vi "RELAYS Delay ON a Relay.vi"(6 "delayed Time ( 2 sec)":dbl=2.0, 8 "error in (no error)":errorcluster, 9 "Relays IDs":T1=3 items=["Relay 1"=3, "Relay 2"=8, "Relay 3"=13, "Relay 4"=18, "Relay 5"=23, "Relay 6"=28, "Relay 7"=33, "Relay 8"=38], 10 "Dev addr":u8=1 format="%x", 11 "VISA resource name":refnum<visa-resource-name>) -> (0 "error out":errorcluster, 1 "success?":bool, 2 "ack":string, 3 "VISA resource name out":refnum<visa-resource-name>)   [LabVIEW 2016, in "MB _relays.lvlib"]
uses:
  MB _relays.lvlib
  type defs/Relays IDs flash.ctl
  private/gen MB frame -Delayed ON Relay.vi
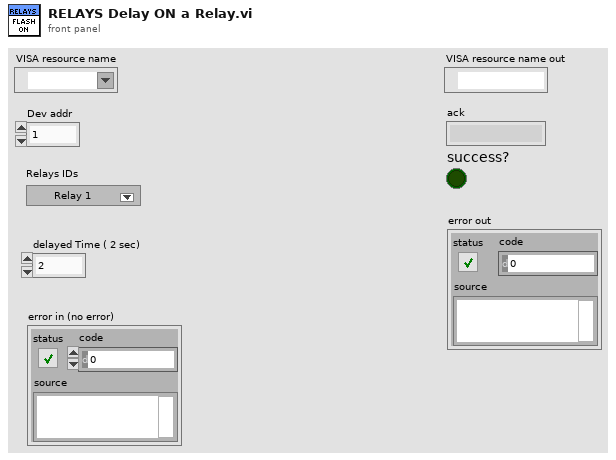
[diagram p1: front panel]
types:
  T1 = typedef "MB _relays.lvlib/Relays IDs flash.ctl" = u16
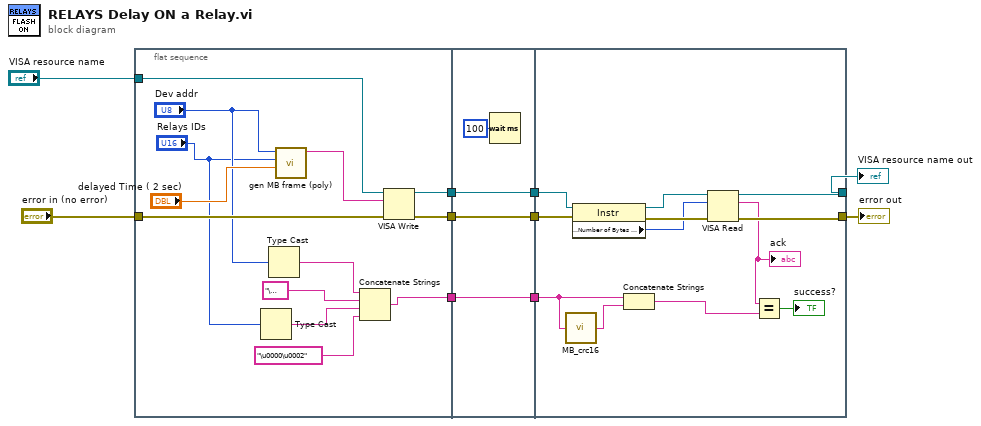
[diagram p0: block diagram]
diagram:
  n1 = flat-sequence {
    tunnel: "error in (no error)" -> [w20]
    tunnel: "VISA resource name" -> [w19]
    tunnel: [w23] -> w6
    tunnel: [w22] -> w5
    tunnel: [w11] -> w2
    tunnel: w6 -> [w27]
    tunnel: w5 -> [w26]
    tunnel: [w27] -> w4
    tunnel: [w26] -> w3
    tunnel: w2 -> [w24]
    tunnel: [w24] -> w1
    tunnel: [w33] -> w9
    tunnel: [w34] -> w10
    tunnel: w4 -> [w38]
    tunnel: w3 -> [w39]
    tunnel: w1 -> [w31]
    frame #0 {
      n2 = Type Cast(x="Relays IDs") -> (*(type *) &x=w13:string)  [unwired: 1 in]
      n3 = Type Cast(x="Dev addr") -> (*(type *) &x=w15:string)  [unwired: 1 in]
      n4 = call-poly "gen MB frame (poly).vi"("Half Period(sec)"="delayed Time ( 2 sec)", "Relays IDs"="Relays IDs", "Dev Addr"="Dev addr") -> ("MB frame"=w21:string)  [unwired: 8 in]
      n5 = Concatenate Strings(w15, "\u0010", w13, "\u0000\u0002") -> (w11:string)
      n6 = VISA Write(VISA resource name=w19, write buffer=w21, error in (no error)=w20) -> (VISA resource name out=w23:refnum<visa-resource-name>, error out=w22:errorcluster)  [unwired: 1 out]
    }
    frame #1 {
      n7 = Wait (ms)(milliseconds to wait=u32 100) -> ()  [unwired: 1 out]
    }
    frame #2 {
      n8 = call "MB_crc16.vi"("message"=w31) -> ("CRC16"=w32:string)  [unwired: 4 in]
      n9 = property class="Instr"(reference=w38, error in=w39) -> (reference out=w36:refnum<visa-resource-name>, error out=w37:errorcluster, "Serial Settings:Number of Bytes at Serial Port"=w35:u32)
      n10 = Concatenate Strings(w31, w32) -> (w29:string)
      n11 = VISA Read(VISA resource name=w36, byte count=w35, error in (no error)=w37) -> (VISA resource name out=w34:refnum<visa-resource-name>, read buffer=w30:string, error out=w33:errorcluster)  [unwired: 1 out]
      "ack" <- w30
      n12 = Equal?(x=w30, y=w29) -> (x = y?=→"success?":bool)
    }
  }
  "VISA resource name out" <- w10
  "error out" <- w9
